vi "100k (SubVI).vi"(1 "Fs":dbl, 2 "Array":dbl[](array[numeric])) -> (0 "Y":dbl[](array[numeric]))   [LabVIEW 2014]
uses:
  <vilib>/addons/Sound and Vibration/svt_Weighting/SVT A, B, C Weighting Filter (Fixed Rates) (1 Ch).vi
  <vilib>/addons/Sound and Vibration/svt_Level/SVL Exp Avg Sound Level (1 Ch).vi
  <vilib>/addons/Sound and Vibration/svt_Level/SoundVib_SoundLevel.lvlib
  <vilib>/addons/Sound and Vibration/svt_Weighting/SoundVib_ABCWeighting.lvlib
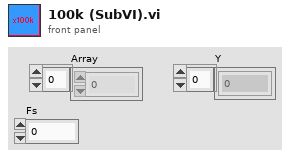
[diagram p1: front panel]
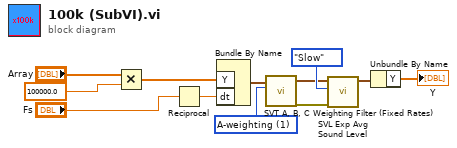
[diagram p0: block diagram]
diagram:
  w10 = u16 1 items=["Linear", "A-weighting", "B-weighting", "C-weighting"] ("weighting")
  n1 = Multiply(x="Array", y=100000.0) -> (x*y=w1:dbl[])
  n2 = Reciprocal(x="Fs") -> (1/x=w5:dbl)
  n3 = Bundle By Name("Y"=w1, "dt"=w5) -> (w6:waveform(dbl))  [unwired: 1 in]
  n4 = call-poly <vilib>:"SVT A, B, C Weighting Filter (Fixed Rates).vi"("weighting"=w10, "scaled signal [EU]"=w6) -> ("error out"=w9:errorcluster, "weighted signal [EU]"=w8:waveform(dbl))  [unwired: 7 in]
  n5 = call-poly <vilib>:"SVL Exp Avg Sound Level.vi"("error in (no error)"=w9, "exponential mode"=enum16{"Slow", "Fast", "Impulse", "Custom"}."Slow", "scaled signal [EU]"=w8) -> ("exp avg sound level [dB EU]"=w7:waveform(dbl))  [unwired: 4 in, 4 out]
  n6 = Unbundle By Name(w7) -> ("Y"=→"Y":dbl[])
